vi "blink.vi"(7 "system state in":T2, 11 "mode set":T1) -> (8 "system state out":T2)   [LabVIEW 2016]
doc: "This subvi just makes the 4 way intersection to blink on and off, very similar when a real 4 way intersaction performs the same tasks.\n\nAlexis Lopez\nP350\nCSUSB Physics"
uses:
  typedefs/system state cluster.ctl
  typedefs/state enum.ctl
  typedefs/control mode enum.ctl
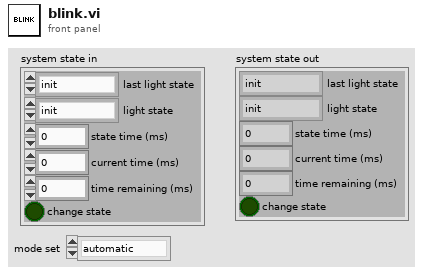
[diagram p1: front panel]
types:
  T1 = typedef "control mode enum.ctl" = enum16{"automatic", "blinking", "all on test"}
  T2 = typedef "system state cluster.ctl" = cluster{"last light state":T3, "light state":T3, "state time (ms)":i32, "current time (ms)":i32, "time remaining (ms)":i32, "change state":bool}
  T3 = typedef "state enum.ctl" = enum16{"init", "idle", "left turn E", "go EW", "caution EW", "left turn W", "left turn N", "go NS", "caution NS", "left turn S", "blink on", "blink off", "all on test", "exit"}
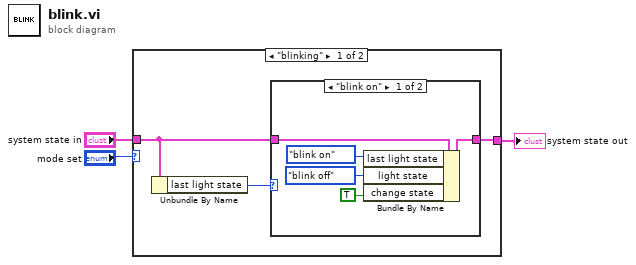
[diagram p0: block diagram]
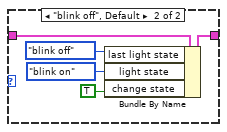
[diagram p2: hidden frame]
diagram:
  n1 = case shown="\"blinking\"" "mode set" {
    tunnel: "system state in" -> [w5 w17]
    tunnel: [w6 w17] -> w2
    frame "blinking" {
      n2 = Unbundle By Name(w5) -> ("last light state"=w4:T3)
      n3 = case shown="\"blink on\"" w4 {
        tunnel: [w11 w15] -> w6
        tunnel: w5 -> [w8 w16]
        frame "blink on" {
          n4 = Bundle By Name(cluster=w8, "last light state"=state_enum."blink on" ("light state"), "light state"=state_enum."blink off", "change state"=TRUE) -> (w11:T2)
        }
        frame "blink off", Default {
          n5 = Bundle By Name(cluster=w16, "last light state"=state_enum."blink off" ("light state"), "light state"=state_enum."blink on", "change state"=TRUE) -> (w15:T2)
        }
      }
    }
    frame "all on test", Default {
    }
  }
  "system state out" <- w2
